vi "mark_finished_missions.vi"(9 "Finished Missions":refnum<class "GenericMission.lvclass">[](array[class]), 10 "Current Missions (human readable)":T1[](array[typedef]) {"Points of Interest"."North" format="%#_10f"; "Points of Interest"."East" format="%#_8f"}, 11 "Current Missions":refnum<class "GenericMission.lvclass">[](array[class])) -> (2 "Current Missions OUT":T1[](array[typedef]) {"Points of Interest"."North" format="%#_10f"; "Points of Interest"."East" format="%#_8f"}, 3 "Current Missions OUT":refnum<class "GenericMission.lvclass">[](array[class]))   [LabVIEW 2013]
doc: "This VI takes in arrays of current missions and finished missions, then goes through the array of finished missions and marks current missions finished if they haven't yet been.\n\nEric Schneider, June 2014"
uses:
  cRIO_Code/Data/TypeDefs/MissionDescription.ctl
  cRIO_Code/Data/TypeDefs/MissionTypeControl.ctl
  cRIO_Code/Data/TypeDefs/UTM Location.ctl
  cRIO_Code/Logic/Classes/Missions/GenericMission/GenericMission.lvclass
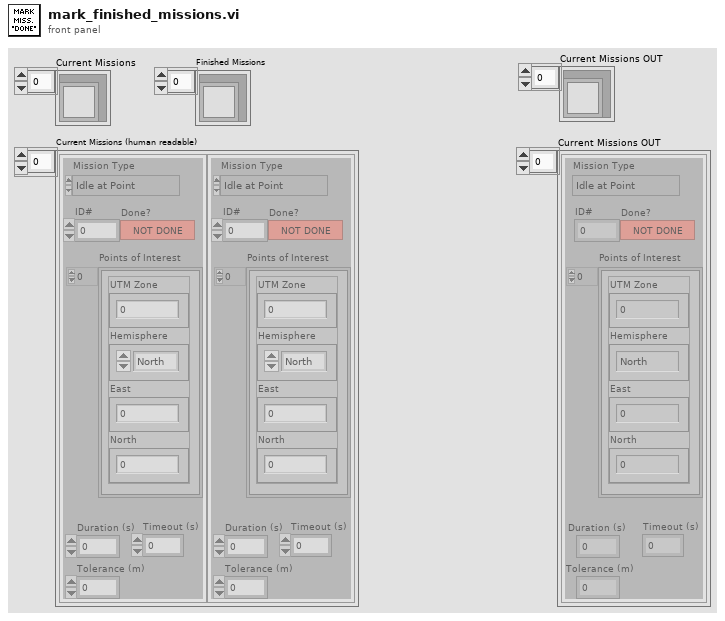
[diagram p1: front panel]
types:
  T1 = typedef "MissionDescription.ctl" = cluster{"Duration (s)":dbl, "Timeout (s)":dbl, "Tolerance (m)":dbl, "Mission Type":T2, "Points of Interest":T3[], "ID#":i32, "Done?":bool}
  T2 = typedef "MissionTypeControl.ctl" = enum16{"Idle at Point", "Drive to Waypoint", "Round Buoy to Port", "Round Buoy to Starboard", "Pass Between Buoys", "Station Keeping"}
  T3 = typedef "UTM Location.ctl" = cluster{"UTM Zone":dbl, "Hemisphere":enum16{"North", "South"}, "East":dbl, "North":dbl}
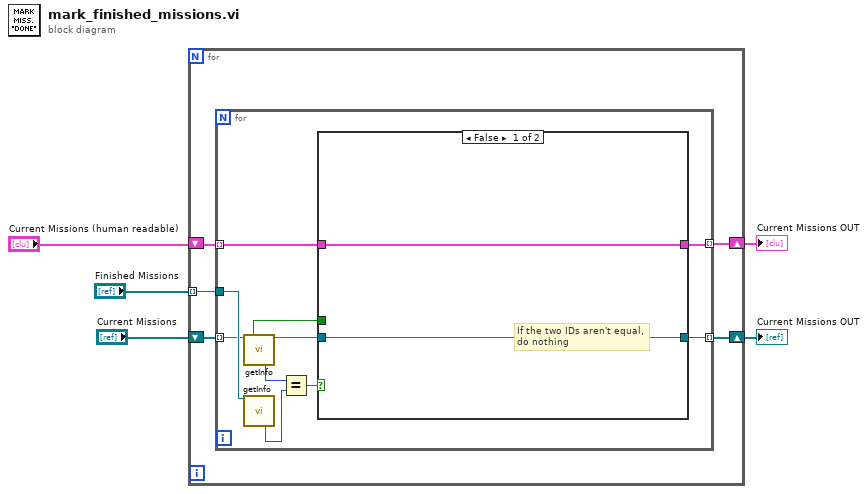
[diagram p0: block diagram]
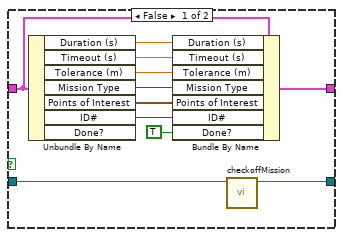
[diagram p3: hidden frame]
diagram:
  n1 = for {
    tunnel: "Finished Missions" -> [w9] mode=indexing
    shift-right: [w7] -> w2
    shift-left: "Current Missions" -> [w10]
    shift-right: [w6] -> w1
    shift-left: "Current Missions (human readable)" -> [w8]
    n2 = for {
      tunnel: w10 -> [w19] mode=indexing
      tunnel: w9 -> [w20]
      tunnel: w8 -> [w16] mode=indexing
      tunnel: [w12] -> w7 mode=indexing
      tunnel: [w11] -> w6 mode=indexing
      n3 = call-dynamic "getInfo.vi"("GenericMission in"=w19) -> ("Done"=w17:bool, "GenericMission out"=w13:refnum<class "GenericMission.lvclass">, "ID#"=w15:i16)  [unwired: 6 in, 6 out]
      n4 = call-dynamic "getInfo.vi"("GenericMission in"=w20) -> ("ID#"=w14:i16)  [unwired: 6 in, 8 out]
      n5 = Equal?(x=w15, y=w14) -> (x = y?=w18:bool)
      n6 = case shown="False" w18 {
        tunnel: w17 -> [_ w27]
        tunnel: w16 -> [w21 w26]
        tunnel: w13 -> [w22 w25]
        tunnel: [w22 w24] -> w12
        tunnel: [w21 w23] -> w11
        frame False {
          # "If the two IDs aren't equal, do nothing"
        }
        frame True {
          n7 = case shown="True" w27 {
            tunnel: w26 -> [w38 w39]
            tunnel: w25 -> [w30 w40]
            tunnel: [w29 w40] -> w24
            tunnel: [w28 w39] -> w23
            frame False {
              n8 = Unbundle By Name(w38) -> ("Duration (s)"=w37:dbl, "Timeout (s)"=w36:dbl, "Tolerance (m)"=w35:dbl, "Mission Type"=w34:T2, "Points of Interest"=w33:T3[], "ID#"=w32:i32)  [unwired: 1 out]
              n9 = Bundle By Name(cluster=w38, "Duration (s)"=w37, "Timeout (s)"=w36, "Tolerance (m)"=w35, "Mission Type"=w34, "Points of Interest"=w33, "ID#"=w32, "Done?"=TRUE) -> (w28:T1)
              n10 = call "checkoffMission.vi"("GenericMission in"=w30) -> ("GenericMission out"=w29:refnum<class "GenericMission.lvclass">)  [unwired: 9 in, 1 out]
            }
            frame True {
              # "If the mission is already marked true, do nothing"
            }
          }
        }
      }
    }
  }
  "Current Missions OUT" <- w2
  "Current Missions OUT" <- w1
